vi "Millisecond timer with error IO.vi"(4 "error in":errorcluster, 5 "T0 time (ms)":u32, 6 "Variant (not connected, use for data flow)":variant) -> (0 "error out":errorcluster, 1 "Elapsed time (ms)":u32, 2 "current millisecond timer value":u32)   [LabVIEW 2013]
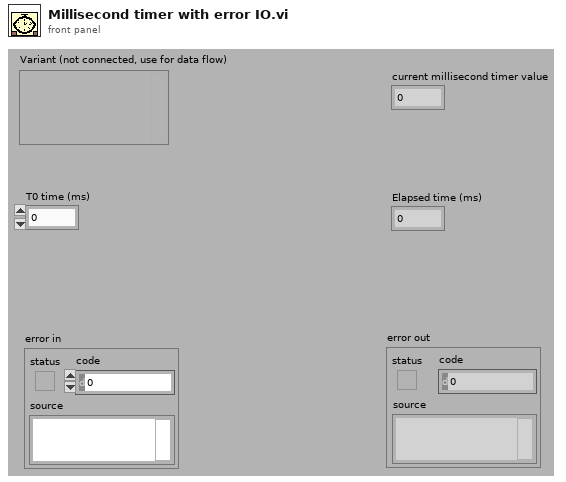
[diagram p1: front panel]
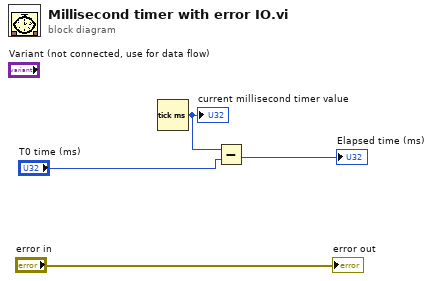
[diagram p0: block diagram]
diagram:
  n1 = Tick Count (ms)() -> (millisecond timer value=w3:u32)
  "current millisecond timer value" <- w3
  n2 = Subtract(x=w3, y="T0 time (ms)") -> (x-y=→"Elapsed time (ms)":u32)
  "error out" <- "error in"
